vi "FTW-Publisher-Publish.vi"(0 "FTW Publisher":refnum<data-value>, 5 "Message":string, 7 "Send Timeout":i32 format="%dmsec", 11 "error in":errorcluster) -> (4 "FTW Publisher out":refnum<data-value>, 15 "error out":errorcluster)   [LabVIEW 2014]
uses:
  core/FTW-Publisher-Core-Type.ctl
  error/FTW-ERR-ThrowGenericError.vi
  error/FTW-ERR-ThrowError.vi
  error/FTW-ERR-NoErrorConstant.vi
  error/FTW-ERR-CallChain.vi
  string/FTW-STR-ReplaceWhitespace.vi
panel:
  # "Inputs"
  # "Outputs"
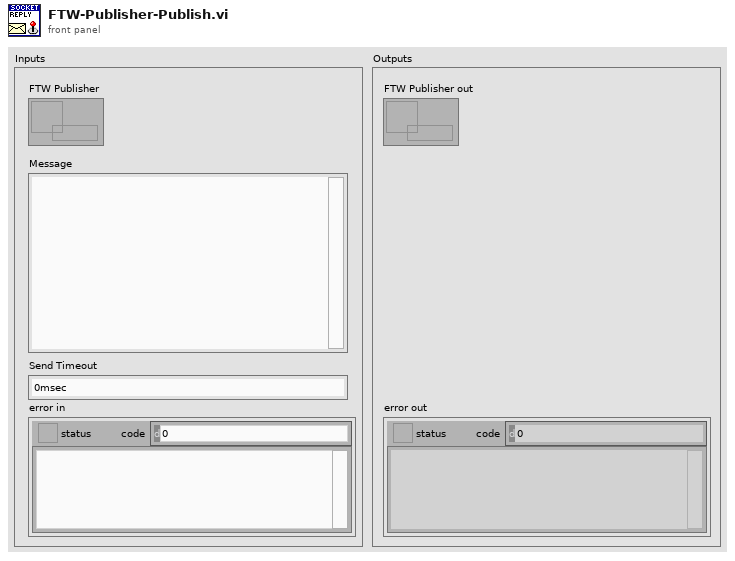
[diagram p1: front panel]
types:
  T1 = typedef "FTW-Publisher-Core-Type.ctl" = cluster{"Socket":i64}
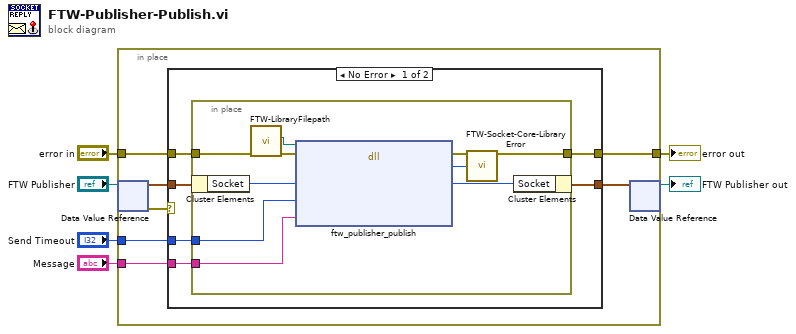
[diagram p0: block diagram]
diagram:
  n1 = in-place {
    in-place-border: "error in" -> [w13]
    in-place-border: [w12] -> w2
    in-place-border: "Send Timeout" -> [w11]
    in-place-border: "Message" -> [w10]
    n2 = in-place-dvr #1("FTW Publisher") -> (w9:T1, w7:errorcluster)
    n3 = case shown="No Error" w7 {
      tunnel: w13 -> [w19 w31]
      tunnel: [w18 w31] -> w12
      tunnel: w11 -> [w17 _]
      tunnel: w10 -> [w16 _]
      tunnel: w9 -> [w15 w30]
      tunnel: [w14 w30] -> w8
      frame No Error {
        n4 = in-place {
          in-place-border: w19 -> [w21]
          in-place-border: [w20] -> w18
          in-place-border: w17 -> [w26]
          in-place-border: w16 -> [w22]
          n5 = in-place-cluster #2(w15) -> ("Socket"=w24:i64)
          n6 = call "FTW-LibraryFilepath.vi"("error in"=w21) -> ("error out"=w27:errorcluster, "Library Filepath"=w28:path)  [unwired: 8 in, 1 out]
          n7 = dll-call lib="?" fn="ftw_publisher_publish"(path in=w28, error in=w27, "Socket"=w24, "Send Timeout"=w26, "Response"=w22) -> (error out=w29:errorcluster, "Return Value"=w25:i64, "Socket"=w23:i64)  [unwired: 3 in, 1 out]
          n8 = call "FTW-Socket-Core-LibraryError.vi"("error in"=w29, "Return Value"=w25) -> ("error out"=w20:errorcluster)  [unwired: 13 in]
          n9 = in-place-cluster #2("Socket"=w23) -> (w14:T1)
        }
      }
      frame Error {
      }
    }
    n10 = in-place-dvr #1(w8) -> (→"FTW Publisher out":refnum<data-value>)  [unwired: 1 out]
  }
  "error out" <- w2
